vi "Load Deployment Hooks.vi"(8 "error in":errorcluster) -> (0 "error out":errorcluster, 3 "Custom Device Deployment Hooks out":refnum<class "Custom Device Deployment Hooks.lvclass">)   [LabVIEW 2026, in "NIDMM Configuration.lvlib"]
uses:
  NIDMM Configuration.lvlib
  <vilib>/Utility/LVLibp/NI_PackedLibraryUtility.lvlib
  <vilib>/Utility/error.llb/whitespace.ctl
  <vilib>/Utility/error.llb/Trim Whitespace (string).vi
  <userlib>/Custom Device Interfaces_v1.lvlibp/CustomDeviceDeploymentHooks/Custom Device Deployment Hooks.lvclass
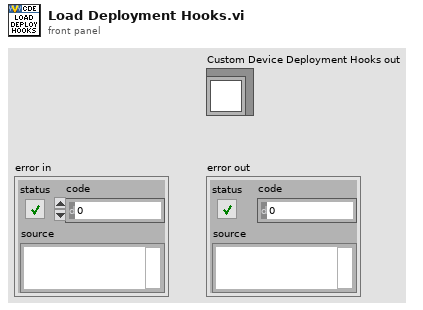
[diagram p1: front panel]
types:
  T1 = typedef "whitespace.ctl" = u16
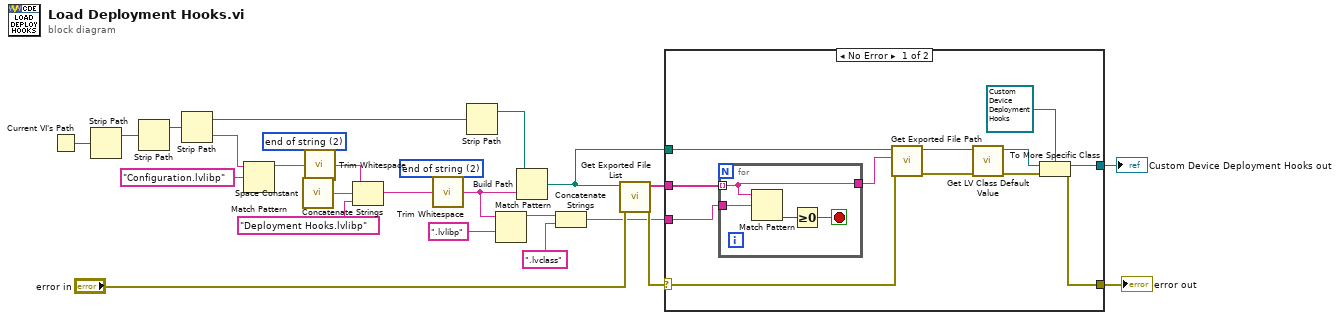
[diagram p0: block diagram]
diagram:
  w9 = T1 2 items=["both", "start of string", "end of string"] ("location (both)")
  w13 = T1 2 items=["both", "start of string", "end of string"] ("location (both)")
  n1 = Current VI's Path() -> (path=w4:path)
  n2 = Strip Path(path=w4) -> (stripped path=w3:path)  [unwired: 1 out]
  n3 = Strip Path(path=w3) -> (stripped path=w2:path)  [unwired: 1 out]
  n4 = Strip Path(path=w2) -> (stripped path=w1:path, name=w16:string)
  n5 = Match Pattern(string=w16, regular expression="Configuration.lvlibp") -> (before substring=w8:string)  [unwired: 1 in, 3 out]
  n6 = call <vilib>:"Space Constant.vi"() -> ("String"=w14:string)
  n7 = call-poly <vilib>:"Trim Whitespace.vi"("string"=w8, "location (both)"=w9) -> ("trimmed string"=w10:string)
  n8 = Concatenate Strings(w10, w14, "Deployment Hooks.lvlibp") -> (w11:string)
  n9 = call-poly <vilib>:"Trim Whitespace.vi"("string"=w11, "location (both)"=w13) -> ("trimmed string"=w7:string)
  n10 = Strip Path(path=w1) -> (stripped path=w12:path)  [unwired: 1 out]
  n11 = Match Pattern(string=w7, regular expression=".lvlibp") -> (before substring=w20:string)  [unwired: 1 in, 3 out]
  n12 = Build Path(base path=w12, name or relative path=w7) -> (appended path=w6:path)
  n13 = Concatenate Strings(w20, ".lvclass" ("regular expression")) -> (w18:string)
  n14 = call <vilib>:"Get Exported File List.vi"("error in (no error)"="error in", "packed library path"=w6) -> ("error out"=w23:errorcluster, "qualified names"=w22:string[])  [unwired: 7 in, 1 out]
  n15 = case shown="No Error" w23 {
    selector: w23 -> [w37 w42]
    tunnel: w22 -> [w33 _]
    tunnel: w6 -> [w32 _]
    tunnel: [w30 _] -> w5
    tunnel: [w36 w42] -> w24
    tunnel: w18 -> [w28 _]
    frame No Error {
      n16 = for {
        tunnel: w33 -> [w38] mode=indexing
        tunnel: w28 -> [w41]
        tunnel: [w38] -> w31
        stop <- w39 stop-if-true
        n17 = Match Pattern(string=w38, regular expression=w41) -> (offset past match=w40:i32)  [unwired: 1 in, 3 out]
        n18 = Greater Or Equal To 0?(x=w40) -> (x >= 0?=w39:bool)
      }
      n19 = call <vilib>:"Get Exported File Path.vi"("error in (no error)"=w37, "qualified name"=w31, "packed library path"=w32) -> ("error out"=w35:errorcluster, "path"=w27:path)  [unwired: 7 in]
      n20 = call <vilib>:"Get LV Class Default Value.vi"("error in (no error)"=w35, "class path"=w27) -> ("error out"=w34:errorcluster, "object"=w29:refnum<class>)  [unwired: 8 in]
      n21 = To More Specific Class(target class=refnum<class "Custom Device Deployment Hooks.lvclass"> refnum ("iCustomDeviceDeploymentHooks"), reference=w29, error in=w34) -> (specific class reference=w30:refnum<class "Custom Device Deployment Hooks.lvclass">, error out=w36:errorcluster)
    }
    frame Error {
    }
  }
  "error out" <- w24
  "Custom Device Deployment Hooks out" <- w5
